vi "saving.vi"(0 "file path (use dialog)":path=path "Z:/11 Setups/04 NOPA TA/01 Data/20211129/test/test", 1 "save type":bool[](array[boolean]), 2 "details":string[](array[string])=["Title", "Author", "Description"], 3 "signal mean":dbl[](array[numeric]), 5 "wavelength":dbl[](array[numeric]), 7 "signal anis (accum.)":dbl[][](array[numeric]), 9 "time delays":dbl[][](array[numeric]), 11 "signal (accum.)":dbl[][](array[numeric]), 12 "raw data":dbl[][][](array[numeric]), 14 "reference mean":dbl[](array[numeric])) -> ()   [LabVIEW 2019]
uses:
  <vilib>/regexp/Match Regular Expression.xnode
panel:
  # "saving ..."
  # "transients"
  # "signal mean"
  # "reference mean"
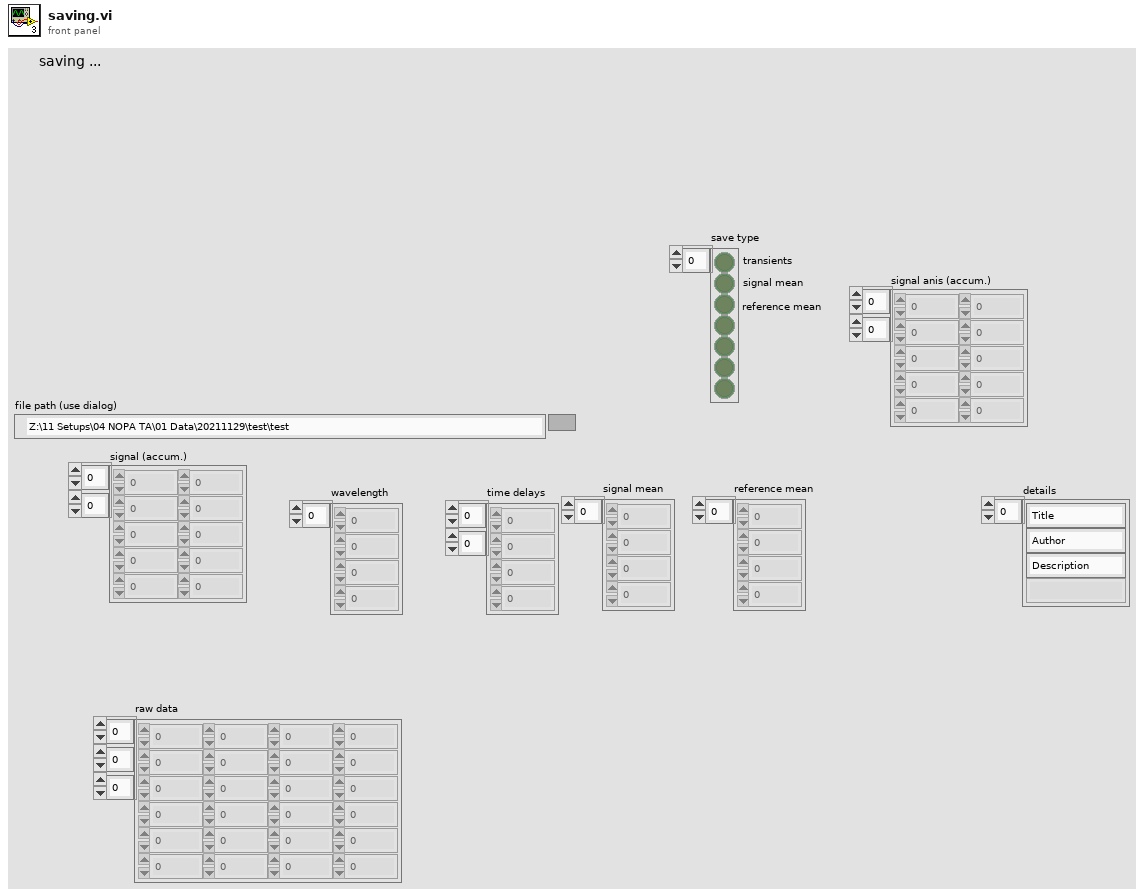
[diagram p1: front panel]
types:
  T1 = enum16{"open", "open or create", "create or replace", "create", "open (read-only)"}
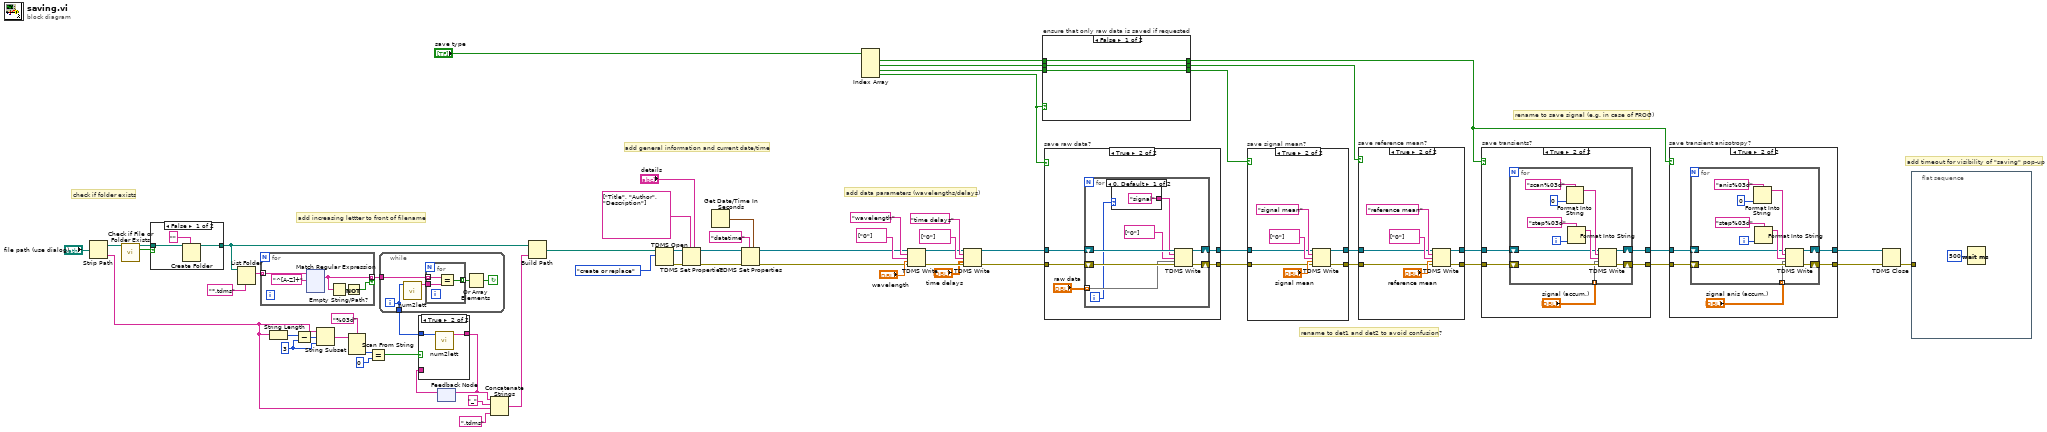
[diagram p0: block diagram]
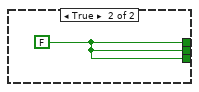
[diagram p3: hidden frame]
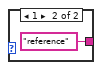
[diagram p5: hidden frame]
diagram:
  w35 = 3
  # "add timeout for visibility of \"saving\" pop-up"
  # "rename to save signal (e.g. in case of FROG)"
  # "rename to det1 and det2 to avoid confusion?"
  # "add data parameters (wavelengths/delays)"
  # "add general information and current date/time"
  # "add increasing lettter to front of filename"
  # "check if folder exists"
  n1 = Strip Path(path="file path (use dialog)") -> (stripped path=w60:path, name=w27:string)
  n2 = call <vilib>:"Check if File or Folder Exists.vi"("path"=w60) -> ("file or folder exists?"=w63:bool, "dup path"=w62:path)  [unwired: 8 in, 1 out]
  n3 = case shown="False" w63 {
    tunnel: [w66 w68] -> w41
    tunnel: w62 -> [w65 w68]
    frame False {
      n4 = Create Folder(prompt (Create Folder)="", path (use dialog)=w65) -> (created path=w66:path)  [unwired: 1 in, 2 out]
    }
    frame True {
    }
  }
  n5 = List Folder(path=w41, pattern="*.tdms") -> (filenames=w40:string[])  [unwired: 2 in, 3 out]
  n6 = for {
    tunnel: w40 -> [w72] mode=indexing
    tunnel: [w71] -> w25 mode=indexing if=w69
    n7 = xnode "Match Regular Expression"("input string"=w72, "regular expression"="^[A-Z]+") -> ("whole match"=w71:string)  [unwired: 4 in, 4 out]
    n8 = Empty String/Path?(string/path=w71) -> (empty?=w70:bool)
    n9 = Not(x=w70) -> (.not. x?=w69:bool)
  }
  n10 = String Length(string=w27) -> (length=w37:i32)
  n11 = Subtract(x=w37, y=w35) -> (x-y=w36:i32)
  n12 = String Subset(string=w27, offset (0)=w36, length (rest)=w35) -> (substring=w34:string)
  n13 = Scan From String(format string="%03d", input string=w34) -> (output 1=w32:i32)  [unwired: 3 in, 3 out]
  n14 = Equal?(x=w32, y=0) -> (x = y?=w30:bool)
  n15 = while {
    tunnel: w25 -> [w192]
    tunnel: [w188] -> w24
    i -> [w188]
    stop <- w189 continue-if-true
    n16 = call "num2lett.vi"("Number"=w188) -> ("Letter"=w191:string)  [unwired: 10 in]
    n17 = for {
      tunnel: w192 -> [w194] mode=indexing
      tunnel: w191 -> [w195]
      tunnel: [w193] -> w190 mode=indexing
      n18 = Equal?(x=w194, y=w195) -> (x = y?=w193:bool)
    }
    n19 = Or Array Elements(Boolean array=w190) -> (logical OR=w189:bool)
  }
  n20 = feedback #1() -> (w28:string)  [unwired: 1 in]
  n21 = case shown="True" w30 {
    tunnel: [w196 w198] -> w26
    tunnel: w28 -> [w196 _]
    tunnel: w24 -> [_ w197]
    frame False {
    }
    frame True {
      n22 = call "num2lett.vi"("Number"=w197) -> ("Letter"=w198:string)  [unwired: 10 in]
    }
  }
  n23 = feedback-in #1(w26) -> ()
  n24 = Concatenate Strings(w26, "_" ("string"), w27, ".tdms" ("string")) -> (w38:string)
  n25 = Build Path(base path=w41, name or relative path=w38) -> (appended path=w43:path)
  n26 = TDMS Open(10:T1."create or replace" ("operation (0:open)"), 11:w43) -> (0:w51:errorcluster, 3:w58:refnum<k34>)  [unwired: 5 in]
  n27 = TDMS Set Properties(5:"details", 7:string[] ["Title", "Author", "Description"] ("property names"), 8:w51, 11:w58) -> (0:w13:errorcluster, 3:w14:refnum<k34>)  [unwired: 2 in, 2 out]
  n28 = Get Date/Time In Seconds() -> (seconds since 1Jan1904=w9:timestamp)
  n29 = TDMS Set Properties(5:w9, 7:"datetime", 8:w13, 11:w14) -> (0:w11:errorcluster, 3:w12:refnum<k34>)  [unwired: 2 in, 2 out]
  n30 = Index Array(array="save type") -> (element #1=w17:bool, element #2=w18:bool, element #3=w20:bool, element #4=w8:bool)  [unwired: 4 in]
  n31 = TDMS Write(0:w12, 5:"wavelength" ("group name in (Untitled)"), 7:string[] ["0"] ("channel name(s) in (Untitled)"), 9:"wavelength", 11:w11) -> (4:w52:refnum<k34>, 15:w50:errorcluster)  [unwired: 1 in, 2 out]
  n32 = TDMS Write(0:w52, 5:"time delays" ("group name in (Untitled)"), 7:string[] ["0"] ("channel name(s) in (Untitled)"), 9:"time delays", 11:w50) -> (4:w22:refnum<k34>, 15:w21:errorcluster)  [unwired: 1 in, 2 out]
  n33 = case "ensure that only raw data is saved if requested" shown="False" w8 {
    tunnel: w20 -> [w199 _]
    tunnel: [w199 w202] -> w19
    tunnel: w18 -> [w200 _]
    tunnel: w17 -> [w201 _]
    tunnel: [w201 w202] -> w1
    tunnel: [w200 w202] -> w16
    frame False {
    }
    frame True {
      w202 = FALSE
    }
  }
  n34 = case "save raw data?" shown="True" w8 {
    tunnel: w22 -> [w204 w209]
    tunnel: [w204 w206] -> w7
    tunnel: [w203 w207] -> w6
    tunnel: w21 -> [w203 w208]
    frame False {
    }
    frame True {
      n35 = for {
        shift-right: [w215] -> w207
        shift-left: w208 -> [w216]
        shift-right: [w214] -> w206
        shift-left: w209 -> [w217]
        tunnel: "raw data" -> [w213] mode=indexing
        i -> [w210]
        n36 = case shown="0, Default" w210 {
          tunnel: ["signal" ("group name in (Untitled)") "reference" ("group name in (Untitled)")] -> w212
          frame 0, Default {
          }
          frame 1 {
          }
        }
        n37 = TDMS Write(0:w217, 5:w212, 7:string[] ["0"] ("channel name(s) in (Untitled)"), 9:w213, 11:w216) -> (4:w214:refnum<k34>, 15:w215:errorcluster)  [unwired: 1 in, 2 out]
      }
    }
  }
  n38 = case "save signal mean?" shown="True" w19 {
    tunnel: w7 -> [w221 w225]
    tunnel: w6 -> [w220 w224]
    tunnel: [w221 w223] -> w47
    tunnel: [w220 w222] -> w46
    frame False {
    }
    frame True {
      n39 = TDMS Write(0:w225, 5:"signal mean" ("group name in (Untitled)"), 7:string[] ["0"] ("channel name(s) in (Untitled)"), 9:"signal mean", 11:w224) -> (4:w223:refnum<k34>, 15:w222:errorcluster)  [unwired: 1 in, 2 out]
    }
  }
  n40 = case "save reference mean?" shown="True" w16 {
    tunnel: w47 -> [w230 w234]
    tunnel: w46 -> [w229 w233]
    tunnel: [w229 w232] -> w45
    tunnel: [w230 w231] -> w44
    frame False {
      # "save reference mean"
    }
    frame True {
      n41 = TDMS Write(0:w234, 5:"reference mean" ("group name in (Untitled)"), 7:string[] ["0"] ("channel name(s) in (Untitled)"), 9:"reference mean", 11:w233) -> (4:w231:refnum<k34>, 15:w232:errorcluster)  [unwired: 1 in, 2 out]
    }
  }
  n42 = case "save transients?" shown="True" w1 {
    tunnel: w44 -> [w239 w244]
    tunnel: w45 -> [w238 w243]
    tunnel: [w239 w242] -> w5
    tunnel: [w238 w241] -> w4
    frame False {
      # "save transient"
    }
    frame True {
      # "save transients"
      n43 = for {
        tunnel: "signal (accum.)" -> [w245] mode=indexing
        shift-right: [w248] -> w242
        shift-left: w244 -> [w250]
        shift-right: [w247] -> w241
        shift-left: w243 -> [w249]
        i -> [w246]
        n44 = Format Into String(format string="scan%03d" ("initial string"), 0) -> (resulting string=w255:string)  [unwired: 2 in, 1 out]
        n45 = Format Into String(format string="step%03d" ("initial string"), w246) -> (resulting string=w251:string)  [unwired: 2 in, 1 out]
        n46 = TDMS Write(0:w250, 5:w255, 7:w251, 9:w245, 11:w249) -> (4:w248:refnum<k34>, 15:w247:errorcluster)  [unwired: 1 in, 2 out]
      }
    }
  }
  n47 = case "save transient anisotropy?" shown="True" w1 {
    tunnel: w5 -> [w257 w262]
    tunnel: w4 -> [w256 w261]
    tunnel: [w257 w260] -> w3
    tunnel: [w256 w259] -> w2
    frame False {
      # "save transient"
    }
    frame True {
      # "save transients"
      n48 = for {
        tunnel: "signal anis (accum.)" -> [w263] mode=indexing
        shift-right: [w266] -> w260
        shift-left: w262 -> [w268]
        shift-right: [w265] -> w259
        shift-left: w261 -> [w267]
        i -> [w264]
        n49 = Format Into String(format string="anis%03d" ("initial string"), 0) -> (resulting string=w273:string)  [unwired: 2 in, 1 out]
        n50 = Format Into String(format string="step%03d" ("initial string"), w264) -> (resulting string=w269:string)  [unwired: 2 in, 1 out]
        n51 = TDMS Write(0:w268, 5:w273, 7:w269, 9:w263, 11:w267) -> (4:w266:refnum<k34>, 15:w265:errorcluster)  [unwired: 1 in, 2 out]
      }
    }
  }
  n52 = TDMS Close(8:w2, 11:w3) -> (0:w29:errorcluster)  [unwired: 1 out]
  n53 = flat-sequence {
    tunnel: w29 -> [_]
    frame #0 {
      n54 = Wait (ms)(milliseconds to wait=u32 500) -> ()  [unwired: 1 out]
    }
  }
